vi "Output.vi"(10 "Msg Output":refnum<class "Msg Output.lvclass">) -> ()   [LabVIEW 2025, in "jettl.lvlib" / "Stop Msg.lvlib" / "Stop Msg Output.lvclass"]
uses:
  Stop Msg Output.lvclass
  Msg Output/Msg Output.lvclass
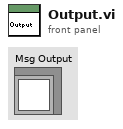
[diagram p1: front panel]
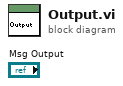
[diagram p0: block diagram]
diagram:
